vi "Turn Off Subpanel Scrollbars When Running.vi"(8 "error in (no error)":errorcluster, 11 "VI":refnum<vi>) -> (0 "error out":errorcluster)   [LabVIEW 2015, in "Utility.lvlib"]
uses:
  Utility.lvlib
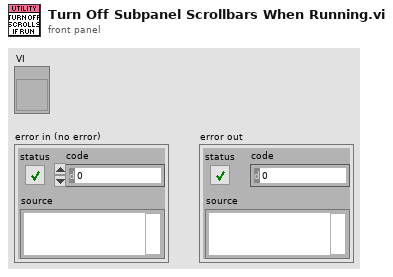
[diagram p1: front panel]
types:
  T1 = enum16{"Always On", "Always Off", "Off While Running"}
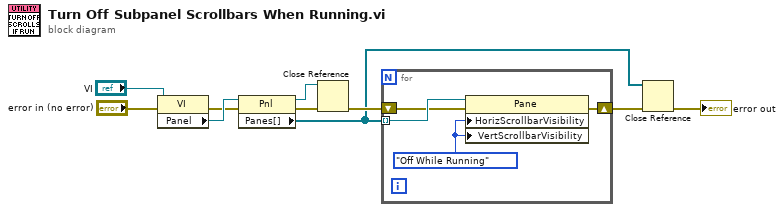
[diagram p0: block diagram]
diagram:
  n1 = property class="VI"(reference="VI", error in="error in (no error)") -> (error out=w6:errorcluster, "Panel"=w7:refnum<vi>)  [unwired: 1 out]
  n2 = property class="Pnl"(reference=w7, error in=w6) -> (reference out=w3:refnum<vi>, error out=w5:errorcluster, "Panes[]"=w1:refnum<vi>[])
  n3 = Close Reference(reference=w3, error in (no error)=w5) -> (error out=w4:errorcluster)
  n4 = for {
    tunnel: w1 -> [w14] mode=indexing
    shift-right: [w11] -> w2
    shift-left: w4 -> [w12]
    w13 = T1."Off While Running" ("Horizontal Scrollbar Visibility")
    n5 = property class="Pane"(reference=w14, error in=w12, "HorizScrollbarVisibility"=w13, "VertScrollbarVisibility"=w13) -> (error out=w11:errorcluster)  [unwired: 1 out]
  }
  n6 = Close Reference(reference=w1, error in (no error)=w2) -> (error out=→"error out":errorcluster)
